vi "Filter FF.vi"(5 "Reset":bool=TRUE, 6 "Elements in buffer":u32, 8 "input valid":bool=TRUE) -> (0 "output valid":bool, 3 "done":bool)   [LabVIEW 2018]
uses:
  <instrlib>/_niInstr/Basic Elements/v1/FPGA/niInstr Basic Elements v1 FPGA.lvlib
  <instrlib>/_niInstr/Basic Elements/v1/FPGA/Private/Count Down U32.vi
  <instrlib>/_niInstr/Basic Elements/v1/FPGA/Private/Count Up U32.vi
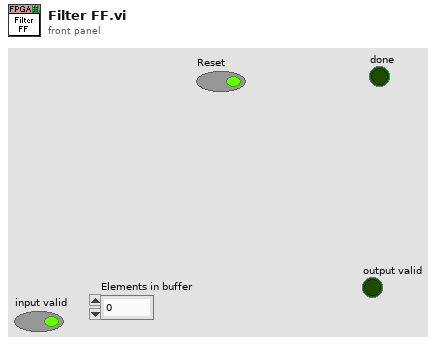
[diagram p1: front panel]
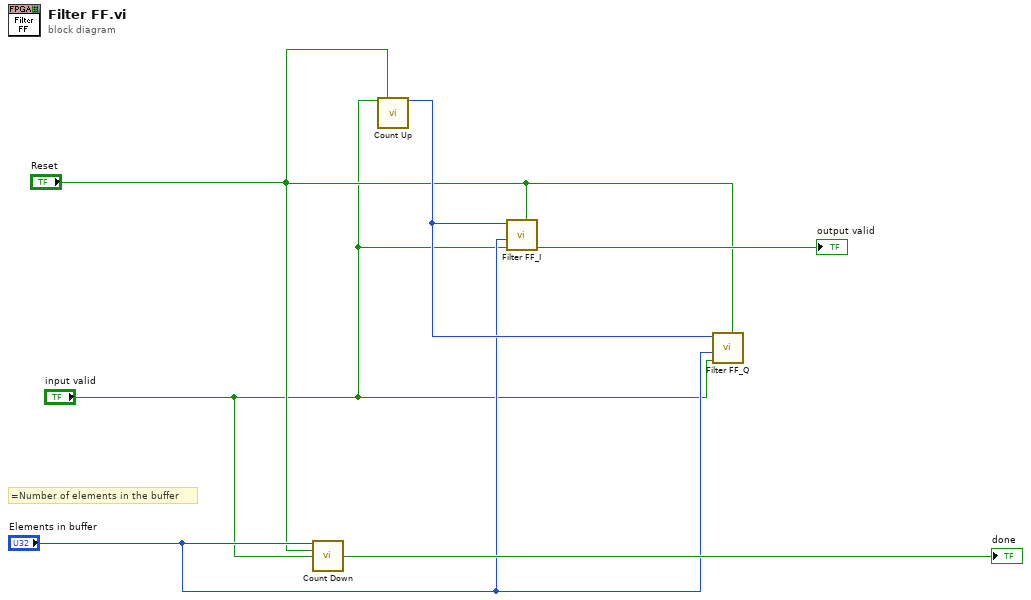
[diagram p0: block diagram]
diagram:
  # "=Number of elements in the buffer"
  n1 = call-poly <instrlib>:"Count Down.vi"("count in"="Elements in buffer", "load"="Reset", "decrement"="input valid") -> ("terminal count"=→"done":bool)  [unwired: 11 in, 1 out]
  n2 = call-poly <instrlib>:"Count Up.vi"("increment"="input valid", "reset"="Reset") -> ("count out"=w4:u32)  [unwired: 13 in]
  n3 = call "Filter FF_I.vi"("Reset"="Reset", "input valid"="input valid", "Buffer size"="Elements in buffer", "source adress"=w4) -> ("output valid"=→"output valid":bool)  [unwired: 7 in]
  n4 = call "Filter FF_Q.vi"("Reset"="Reset", "input valid"="input valid", "Buffer size"="Elements in buffer", "source adress"=w4) -> ()  [unwired: 7 in, 1 out]
